vi "Write Shutter IO Lines.vi"(8 "error in (no error)":errorcluster, 10 "Shutter IO Lines":tag[](array[tag]), 11 "Uniblitz Shutter in":refnum<class "Uniblitz Shutter.lvclass">) -> (0 "error out":errorcluster, 3 "Uniblitz Shutter out":refnum<class "Uniblitz Shutter.lvclass">)   [LabVIEW 2015]
uses:
  Uniblitz Shutter.lvclass
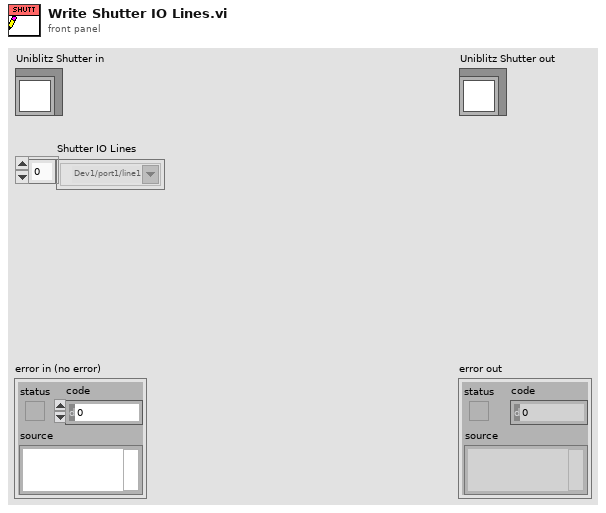
[diagram p1: front panel]
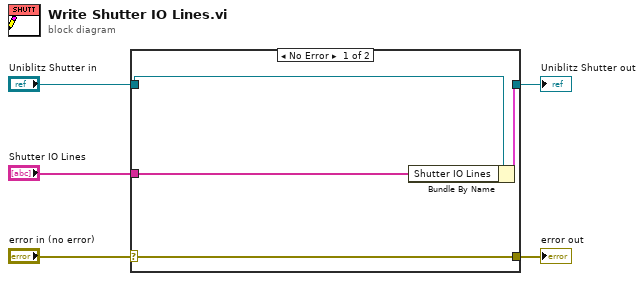
[diagram p0: block diagram]
diagram:
  n1 = case shown="No Error" "error in (no error)" {
    selector: "error in (no error)" -> [w9 w10]
    tunnel: [w9 w10] -> w4
    tunnel: [w7 w11] -> w2
    tunnel: "Uniblitz Shutter in" -> [w8 w11]
    tunnel: "Shutter IO Lines" -> [w6 _]
    frame No Error {
      n2 = Bundle By Name(cluster=w8, "Shutter IO Lines"=w6) -> (w7:cluster{})
    }
    frame Error {
    }
  }
  "error out" <- w4
  "Uniblitz Shutter out" <- w2
